vi "VG_DRIVE.vi"() -> ()   [LabVIEW 2020]
panel:
  out "DRIVE":bool
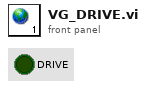
[diagram p1: front panel]
diagram:
